vi "Convert Measurement.vi"() -> ()   [LabVIEW 2021]
uses:
  _Measurement Plugin Converter/Converter/Queue Driver/controls/Queue Operations.ctl
  _Measurement Plugin Converter/Converter/Conversion Logic/controls/Data Holder.ctl
  _Measurement Plugin Converter/Converter/Conversion Logic/controls/Input Data.ctl
  _Measurement Plugin Converter/Converter/Conversion Logic/controls/Module Data.ctl
  _Measurement Plugin Converter/Utilities/Logger Utilities/Event Logger/TypeDef/EventDataCluster.ctl
  _Measurement Plugin Converter/Utilities/Logger Utilities/Event Logger/TypeDef/EventValues.ctl
  _Measurement Plugin Converter/Converter/Converter Reusables/controls/Dictionary States.ctl
  <vilib>/Utility/cursorutil.llb/Set Cursor (Icon Pict).vi
  _Measurement Plugin Converter/Converter/Queue Driver/Queue Driver.lvlib
  _Measurement Plugin Converter/Converter/Conversion Logic/Converter.lvlib
  _Measurement Plugin Converter/Converter/Path Functions/Path Functions.lvlib
  _Measurement Plugin Converter/Converter/Converter Reusables/Converter Reusables.lvlib
  _Measurement Plugin Converter/Utilities/Logger Utilities/Event Logger/Event Logger.lvlib
  _Measurement Plugin Converter/Utilities/Sequence Creation/Create Sequence.lvlib
panel:
  out "Tab Control":enum32{"User Inputs", "Progress", "Next Steps"}(tab)
  in  "CreateSeq?":bool
  in  "Description":string caption="Measurement Plug-in Description"
  in  "Project Path":path caption="Select the Project Path"
  in  "Measurement VI":path caption="Select Measurement VI"
  in  "Plug-in Name":string caption="Measurement Plug-in Name"
  in  "Create Measurement Service":bool
  out "Warning":bool=TRUE caption="1. Measurement should be a VI\n2. Measurement plug-in name must be unique \n3. Plugin name cannot contain any of the following characters:\n         \\ / : * ? \" < > |"
  out "Progress":i8(slide) scale=0.0..100.0
  out "Status":string
  in  "Go Home":bool
  out "Launch IS":string
  out "Run Service":string
  out "Launch Type Spec":string
  out "Launch Logic":string
  out "Launch UI":string
  out "Pinmap Link":string
  out "TestStand Link":string
  out "MeasLink Link":string
  # "* Project in which the measurement plug-in will be created"
  # "Measurement Converted Successfully!"
  # "Run the Measurement:\n1. Run the measurement service. Click here to run.\n2. Launch the Template InstrumentStudio project.\n3. Add instruments and pins in PinMap.\n4. Add SoftPanel and run the measurement."
  # "Review the Measurement:\n1. Review the Measurement UI. Click here to launch.\n2. Review the Measurement Logic VI. Click here to launch.\n3. Review the Type Specialization VI. Click here to launch."
  # "Related Information:\n• InstrumentStudio Pro\n• PinMap\n• TestStand"
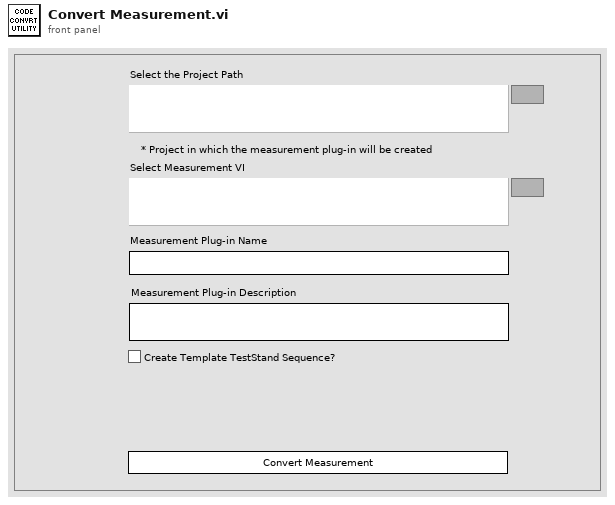
[diagram p1: front panel]
types:
  T1 = typedef "Queue Driver.lvlib/Queue Operations.ctl" = enum16{"Create Q", "Enqueue", "Enqueue N", "Dequeue", "Flush", "Release"}
  T2 = enum8{"Enabled", "Disabled", "Disabled and Grayed Out"}
  T3 = typedef "Converter.lvlib/Data Holder.ctl" = cluster{"Input Data":T4, "Module Data":T5, "TestStandAval?":bool, "EventData":T6}
  T4 = typedef "Converter.lvlib/Input Data.ctl" = cluster{"Project Path":path, "Code Module":path, "Measurement Name":string, "Description":string, "CreateSeq?":bool}
  T5 = typedef "Converter.lvlib/Module Data.ctl" = cluster{"Valid Code Path?":bool, "Valid Meas Name?":bool, "VI extension":string}
  T6 = typedef "Event Logger.lvlib/EventDataCluster.ctl" = cluster{"LoggerPath":path, "FileCount":i32, "EventValues":T7, "ExtendedFilePath":path}
  T7 = typedef "Event Logger.lvlib/EventValues.ctl" = string
  T8 = typedef "Converter Reusables.lvlib/Dictionary States.ctl" = enum16{"Set", "Get", "Delete", "Delete All"}
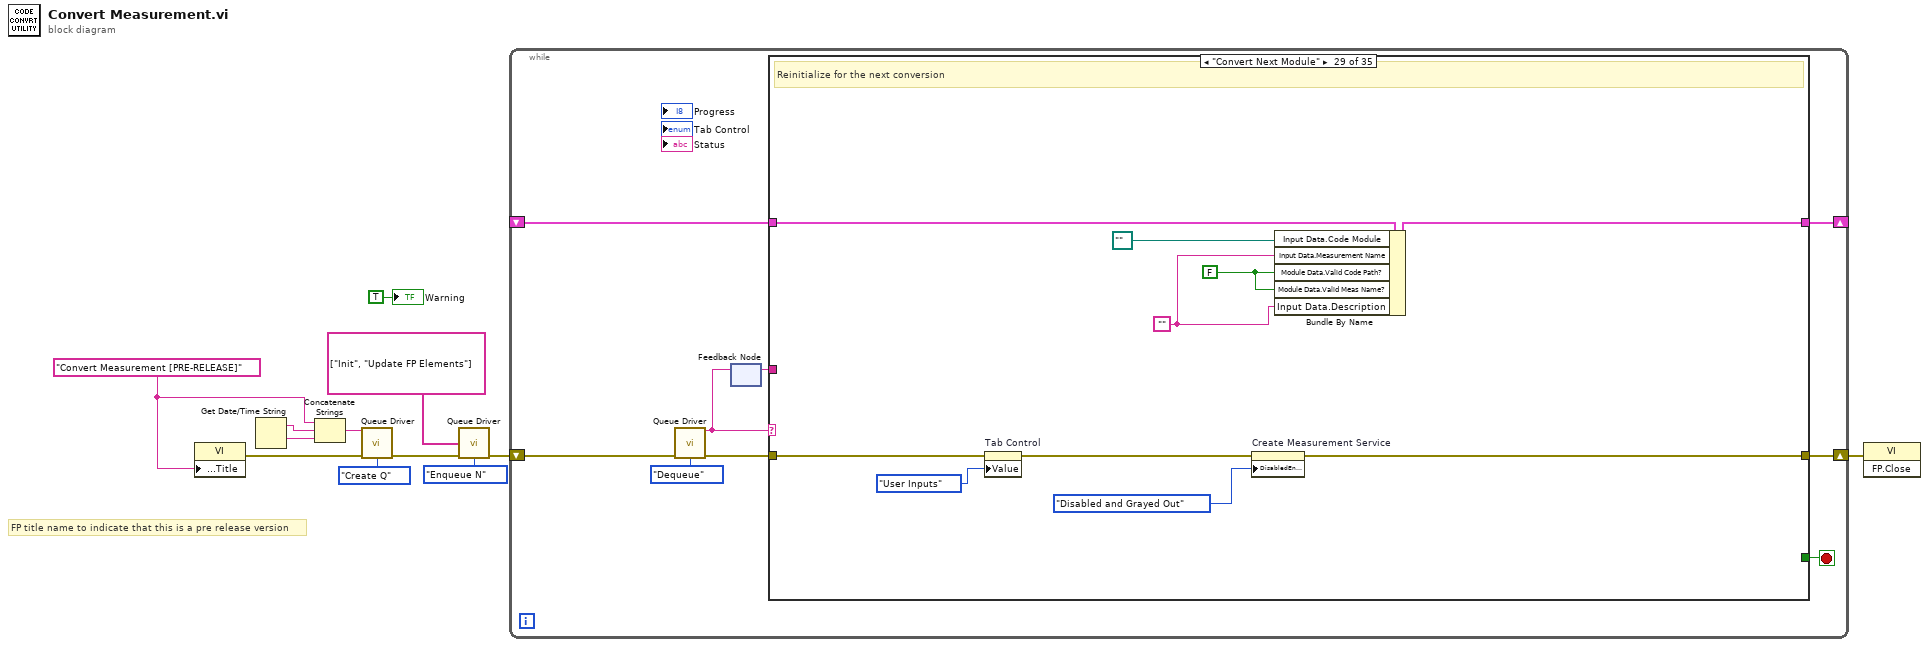
[diagram p0: block diagram]
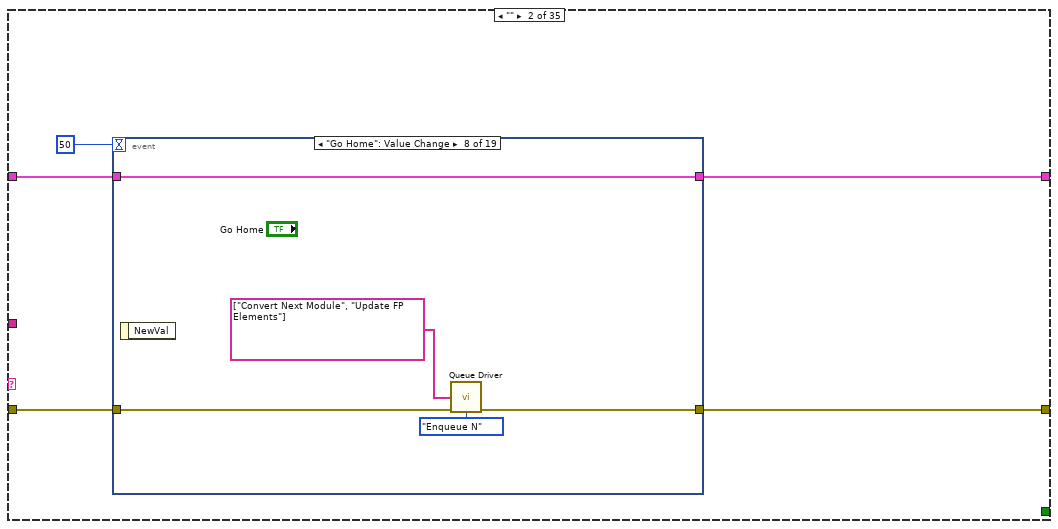
[diagram p3: hidden frame]
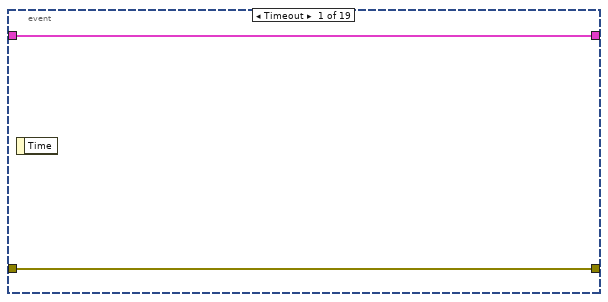
[diagram p4: hidden frame]
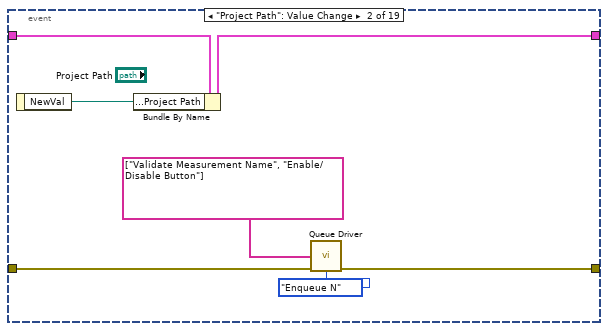
[diagram p5: hidden frame]
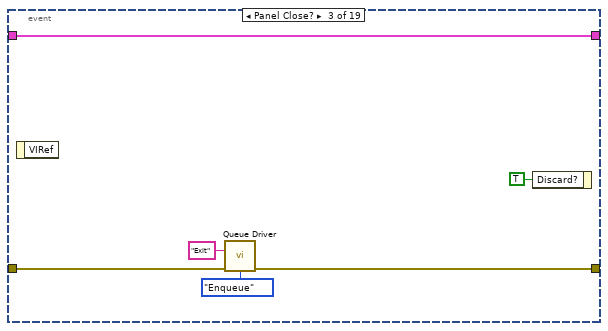
[diagram p6: hidden frame]
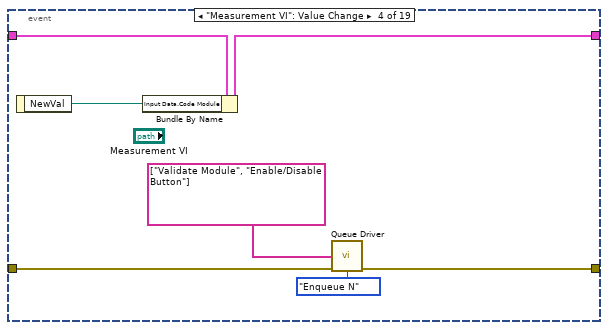
[diagram p7: hidden frame]
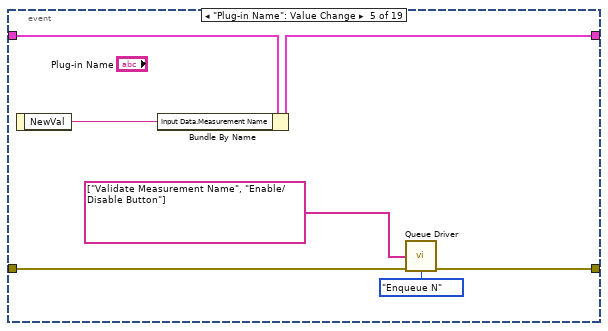
[diagram p8: hidden frame]
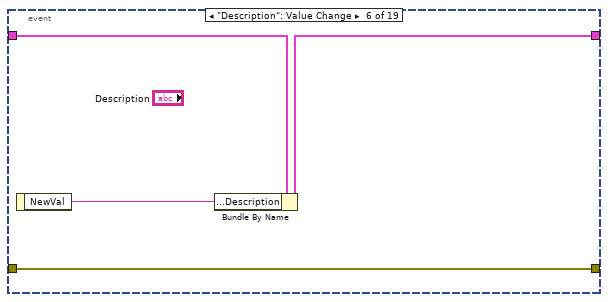
[diagram p9: hidden frame]
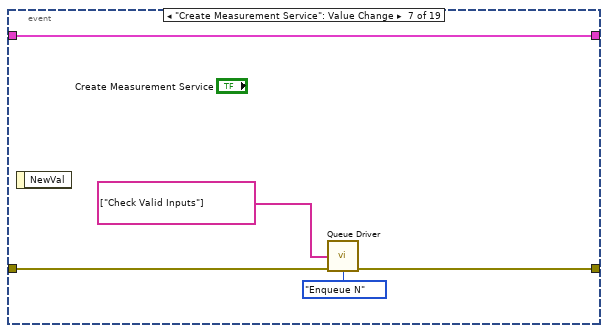
[diagram p10: hidden frame]
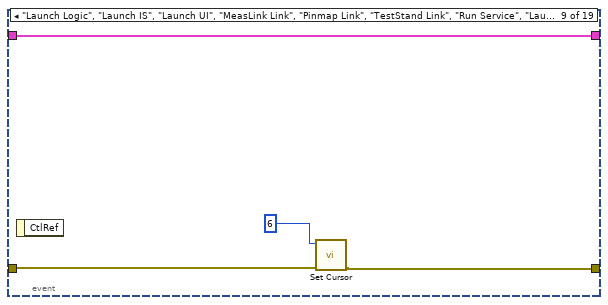
[diagram p11: hidden frame]
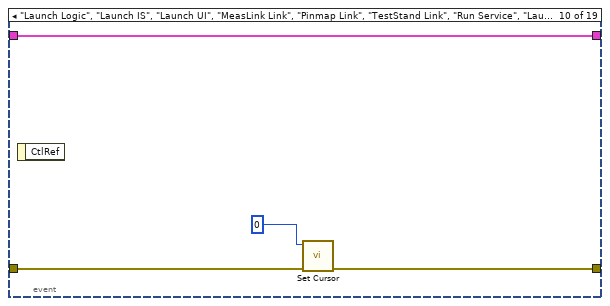
[diagram p12: hidden frame]
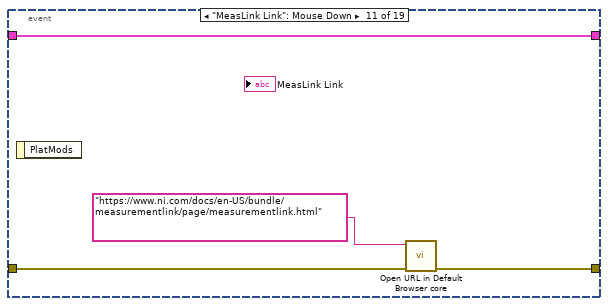
[diagram p13: hidden frame]
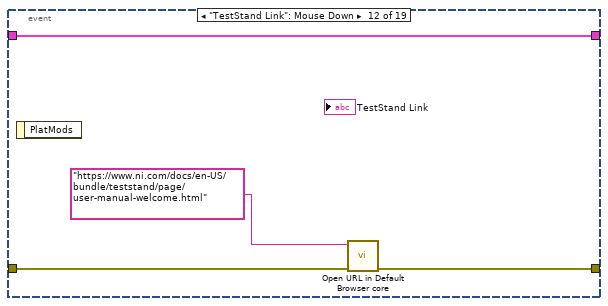
[diagram p14: hidden frame]
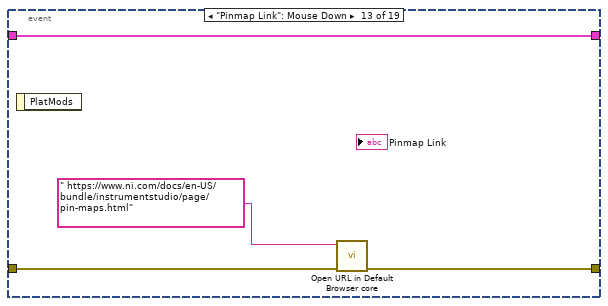
[diagram p15: hidden frame]
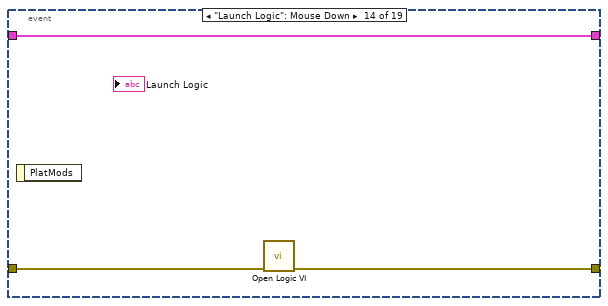
[diagram p16: hidden frame]
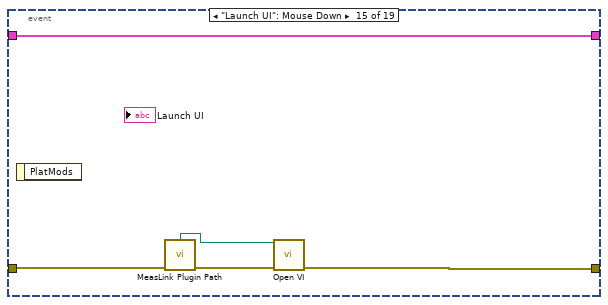
[diagram p17: hidden frame]
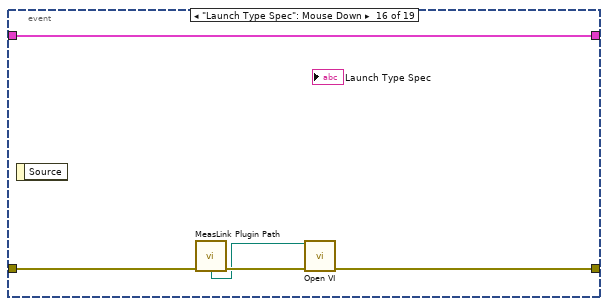
[diagram p18: hidden frame]
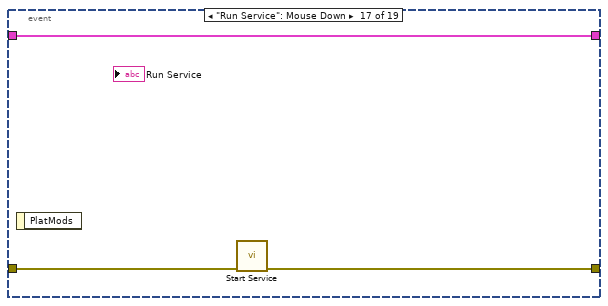
[diagram p19: hidden frame]
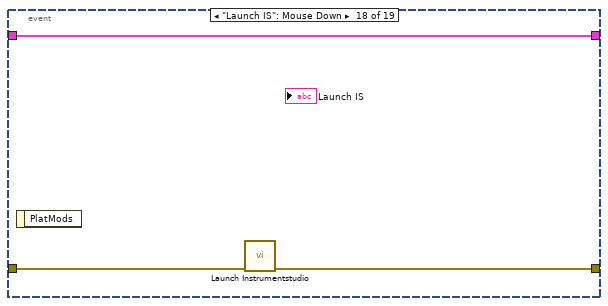
[diagram p20: hidden frame]
diagram:
  w1 = "Convert Measurement [PRE-RELEASE]" ("Front Panel Window:Title")
  # "FP title name to indicate that this is a pre release version"
  n1 = property class="VI"("Front Panel.Title"=w1) -> (error out=w2:errorcluster)  [unwired: 2 in, 1 out]
  n2 = Get Date/Time String() -> (date string=w8:string, time string=w7:string)  [unwired: 3 in]
  n3 = Concatenate Strings(w1, w8, w7) -> (w6:string)
  n4 = call "Queue Driver.vi"("Name"=w6, "error in (no error)"=w2, "Q Operations"=Queue_Operations."Create Q") -> ("error out"=w9:errorcluster)  [unwired: 11 in, 1 out]
  n5 = call "Queue Driver.vi"("States[]"=string[] ["Init", "Update FP Elements"], "error in (no error)"=w9, "Q Operations"=Queue_Operations."Enqueue N") -> ("error out"=w11:errorcluster)  [unwired: 11 in, 1 out]
  n6 = while {
    shift-right: [w18] -> w3
    shift-left: w11 -> [w20]
    shift-right: [w14] -> _
    shift-left: _ -> [w13]
    stop <- w17 stop-if-true
    n7 = call "Queue Driver.vi"("error in (no error)"=w20, "Q Operations"=Queue_Operations."Dequeue") -> ("Dequeued State"=w16:string, "error out"=w19:errorcluster)  [unwired: 12 in]
    n8 = feedback-in #1(w16) -> ()
    n9 = feedback #1() -> (w15:string)  [unwired: 1 in]
    n10 = case shown="\"Convert Next Module\"" w16 {
      tunnel: w19 -> [w23 w27 w132 w134 w146 w156 w161 w165 w188 w212 w223 w231 w245 w254 w263 w275 w285 w297 w306 w318 w329 w339 w350 w361 w373 w384 w404 w426 w437 w443 w449 w451 w459 w462 w464]
      tunnel: [w23 w26 w125 w134 w136 w151 w161 w166 w193 w211 w223 w235 w240 w253 w261 w272 w283 w294 w301 w313 w326 w337 w346 w357 w372 w383 w394 w428 w435 w443 w448 w451 w453 w462 w469] -> w18
      tunnel: [_ _ _ _ _ _ _ _ _ _ _ _ _ _ _ _ _ _ _ _ _ _ _ _ _ _ _ _ _ _ _ _ TRUE _ _] -> w17
      tunnel: w15 -> [_ _ _ _ _ _ _ _ _ _ _ _ _ _ _ _ _ _ _ _ _ _ _ _ _ _ _ _ _ _ _ _ _ _ _]
      tunnel: [w22 w25 w131 w133 w145 w159 w160 w169 w190 w216 w222 w237 w239 w252 w260 w269 w279 w290 w305 w315 w324 w335 w349 w360 w368 w380 w395 w431 w440 w442 w445 w450 w455 w461 w468] -> w14
      tunnel: w13 -> [w22 w24 _ w133 w145 w159 w160 w170 w191 w216 w222 w237 w248 w258 w267 w268 w280 w291 w311 w316 w333 w344 w355 w366 w369 w381 w403 w431 w441 w442 w447 w450 w455 w461 w468]
      frame Default {
      }
      frame "" {
        n11 = event shown="[7] \"Go Home\": Value Change" {
          selector: _ -> [_ _ _ _ _ _ _ _ _ _ _ _ _ _ _ _ _ _ _]
          dyn-events: _ -> [_ _ _ _ _ _ _ _ _ _ _ _ _ _ _ _ _ _ _]
          timeout: 50 -> [_ _ _ _ _ _ _ _ _ _ _ _ _ _ _ _ _ _ _]
          tunnel: w27 -> [w30 w32 w41 w46 w53 w61 w64 w69 w72 w76 w80 w85 w88 w92 w95 w100 w105 w108 w114]
          tunnel: [w30 w33 w40 w45 w54 w61 w65 w70 w73 w77 w81 w86 w89 w93 w96 w101 w106 w109 w114] -> w26
          tunnel: [w29 w36 w43 w49 w56 w59 w66 w71 w75 w79 w83 w87 w91 w94 w99 w104 w107 w110 w112] -> w25
          tunnel: w24 -> [w29 w37 w43 w50 w57 w60 w66 w71 w75 w79 w83 w87 w91 w94 w99 w104 w107 w110 w113]
          event Timeout {
            n12 = event-data() -> ()  [unwired: 1 in, 1 out]
          }
          event "Project Path": Value Change {
            n13 = event-data() -> ("NewVal"=w35:path)  [unwired: 1 in]
            n14 = Bundle By Name(cluster=w37, "Input Data.Project Path"=w35) -> (w36:T3)
            n15 = call "Queue Driver.vi"("States[]"=string[] ["Validate Measurement Name", "Enable/Disable Button"], "error in (no error)"=w32, "Q Operations"=Queue_Operations."Enqueue N") -> ("error out"=w33:errorcluster)  [unwired: 11 in, 1 out]
          }
          event Panel Close? {
            n16 = event-data() -> ()  [unwired: 1 in, 1 out]
            n17 = call "Queue Driver.vi"("State"="Exit", "error in (no error)"=w41, "Q Operations"=Queue_Operations."Enqueue") -> ("error out"=w40:errorcluster)  [unwired: 11 in, 1 out]
            n18 = event-data("Discard?"=TRUE) -> ()  [unwired: 1 in, 1 out]
          }
          event "Measurement VI": Value Change {
            n19 = event-data() -> ("NewVal"=w48:path)  [unwired: 1 in]
            n20 = Bundle By Name(cluster=w50, "Input Data.Code Module"=w48) -> (w49:T3)
            n21 = call "Queue Driver.vi"("States[]"=string[] ["Validate Module", "Enable/Disable Button"], "error in (no error)"=w46, "Q Operations"=Queue_Operations."Enqueue N") -> ("error out"=w45:errorcluster)  [unwired: 11 in, 1 out]
          }
          event "Plug-in Name": Value Change {
            n22 = event-data() -> ("NewVal"=w55:string)  [unwired: 1 in]
            n23 = Bundle By Name(cluster=w57, "Input Data.Measurement Name"=w55) -> (w56:T3)
            n24 = call "Queue Driver.vi"("States[]"=string[] ["Validate Measurement Name", "Enable/Disable Button"], "error in (no error)"=w53, "Q Operations"=Queue_Operations."Enqueue N") -> ("error out"=w54:errorcluster)  [unwired: 11 in, 1 out]
          }
          event "Description": Value Change {
            n25 = event-data() -> ("NewVal"=w58:string)  [unwired: 1 in]
            n26 = Bundle By Name(cluster=w60, "Input Data.Description"=w58) -> (w59:T3)
          }
          event "Create Measurement Service": Value Change {
            n27 = event-data() -> ()  [unwired: 1 in, 1 out]
            n28 = call "Queue Driver.vi"("States[]"=string[] ["Check Valid Inputs"], "error in (no error)"=w64, "Q Operations"=Queue_Operations."Enqueue N") -> ("error out"=w65:errorcluster)  [unwired: 11 in, 1 out]
          }
          event "Go Home": Value Change {
            n29 = event-data() -> ()  [unwired: 1 in, 1 out]
            n30 = call "Queue Driver.vi"("States[]"=string[] ["Convert Next Module", "Update FP Elements"], "error in (no error)"=w69, "Q Operations"=Queue_Operations."Enqueue N") -> ("error out"=w70:errorcluster)  [unwired: 11 in, 1 out]
          }
          event "Launch Logic", "Launch IS", "Launch UI", "MeasLink Link", "Pinmap Link", "TestStand Link", "Run Service", "Launch Type Spec": Mouse Enter {
            n31 = event-data() -> ()  [unwired: 1 in, 1 out]
            n32 = call-poly <vilib>:"Set Cursor.vi"("error in (no error)"=w72, "icon"=u16 6) -> ("error out"=w73:errorcluster)  [unwired: 8 in, 1 out]
          }
          event "Launch Logic", "Launch IS", "Launch UI", "MeasLink Link", "Pinmap Link", "TestStand Link", "Run Service", "Launch Type Spec": Mouse Leave {
            n33 = event-data() -> ()  [unwired: 1 in, 1 out]
            n34 = call-poly <vilib>:"Set Cursor.vi"("error in (no error)"=w76, "icon"=u16 0) -> ("error out"=w77:errorcluster)  [unwired: 8 in, 1 out]
          }
          event "MeasLink Link": Mouse Down {
            n35 = event-data() -> ()  [unwired: 1 in, 1 out]
            n36 = call <vilib>:"Open URL in Default Browser core.vi"("error in (no error)"=w80, "url"="https://www.ni.com/docs/en-US/bundle/measurementlink/page/measurementlink.html" ("URL")) -> ("error out"=w81:errorcluster)  [unwired: 4 in, 1 out]
          }
          event "TestStand Link": Mouse Down {
            n37 = event-data() -> ()  [unwired: 1 in, 1 out]
            n38 = call <vilib>:"Open URL in Default Browser core.vi"("error in (no error)"=w85, "url"="https://www.ni.com/docs/en-US/bundle/teststand/page/user-manual-welcome.html" ("URL")) -> ("error out"=w86:errorcluster)  [unwired: 4 in, 1 out]
          }
          event "Pinmap Link": Mouse Down {
            n39 = event-data() -> ()  [unwired: 1 in, 1 out]
            n40 = call <vilib>:"Open URL in Default Browser core.vi"("error in (no error)"=w88, "url"=" https://www.ni.com/docs/en-US/bundle/instrumentstudio/page/pin-maps.html" ("URL")) -> ("error out"=w89:errorcluster)  [unwired: 4 in, 1 out]
          }
          event "Launch Logic": Mouse Down {
            n41 = event-data() -> ()  [unwired: 1 in, 1 out]
            n42 = call "Open Logic VI.vi"("error in (no error)"=w92) -> ("error out"=w93:errorcluster)  [unwired: 14 in]
          }
          event "Launch UI": Mouse Down {
            n43 = event-data() -> ()  [unwired: 1 in, 1 out]
            n44 = call "MeasLink Plugin Path.vi"("error in (no error)"=w95) -> ("Measurement UI"=w97:path, "error out"=w98:errorcluster)  [unwired: 2 in, 11 out]
            n45 = call "Open VI.vi"("Logic VI Path"=w97, "error in (no error)"=w98) -> ("error out"=w96:errorcluster)  [unwired: 13 in]
          }
          event "Launch Type Spec": Mouse Down {
            n46 = event-data() -> ()  [unwired: 1 in, 1 out]
            n47 = call "MeasLink Plugin Path.vi"("error in (no error)"=w100) -> ("Type Specialization"=w102:path, "error out"=w103:errorcluster)  [unwired: 2 in, 11 out]
            n48 = call "Open VI.vi"("Logic VI Path"=w102, "error in (no error)"=w103) -> ("error out"=w101:errorcluster)  [unwired: 13 in]
          }
          event "Run Service": Mouse Down {
            n49 = event-data() -> ()  [unwired: 1 in, 1 out]
            n50 = call "Start Service.vi"("error in (no error)"=w105) -> ("error out"=w106:errorcluster)  [unwired: 14 in]
          }
          event "Launch IS": Mouse Down {
            n51 = event-data() -> ()  [unwired: 1 in, 1 out]
            n52 = call "Launch Instrumentstudio.vi"("error in (no error)"=w108) -> ("error out"=w109:errorcluster)  [unwired: 14 in]
          }
          event "CreateSeq?": Value Change {
            n53 = event-data() -> ("NewVal"=w111:bool)  [unwired: 1 in]
            n54 = Bundle By Name(cluster=w113, "Input Data.CreateSeq?"=w111) -> (w112:T3)
          }
        }
      }
      frame "Init" {
        # "Initilialize the Data and the UI Data"
        n55 = call "Get Default Project Path.vi"("error in"=w132) -> ("Project Path"=w130:path, "error out"=w128:errorcluster)  [unwired: 13 in]
        n56 = property on="Warning" class="Bool"(error in=w128, "Visible"=FALSE) -> (error out=w126:errorcluster)  [unwired: 1 in, 1 out]
        n57 = property on="Create Measurement Service" class="Bool"(error in=w126, "DisabledEnum"=T2."Disabled and Grayed Out" ("Disabled")) -> (error out=w123:errorcluster)  [unwired: 1 in, 1 out]
        n58 = call "VerifyTestStandAvailability.vi"("Error In"=w123) -> ("TestStandInstalled?"=w116:bool, "Error Out"=w122:errorcluster)  [unwired: 13 in]
        n59 = call "CreateLogFile.vi"("Error In"=w122) -> ("EventDataOut"=w117:T6, "Error Out"=w124:errorcluster)  [unwired: 13 in]
        n60 = property on="CreateSeq?" class="Bool (strict)"(error in=w124, "Value"=w116) -> (error out=w125:errorcluster)  [unwired: 1 in, 1 out]
        n61 = Bundle By Name(cluster=T3 {"Input Data"={"Project Path"=path "", "Code Module"=path "", "Measurement Name"="", "Description"="", "CreateSeq?"=FALSE}, "Module Data"={"Valid Code Path?"=FALSE, "Valid Meas Name?"=FALSE, "VI extension"=""}, "TestStandAval?"=FALSE, "EventData"={"LoggerPath"=path "", "FileCount"=0, "EventValues"="", "ExtendedFilePath"=path ""}} ("Data Holder"), "Input Data.Project Path"=w130, "Input Data.Code Module"=path "", "Input Data.Measurement Name"="", "Module Data.VI extension"="vi" ("Input Data.Measurement Name"), "TestStandAval?"=w116, "Input Data.CreateSeq?"=w116, "EventData"=w117, "Input Data.Description"="") -> (w131:T3)
      }
      frame "*********************FRONT PANEL RELATED****************" {
      }
      frame "Update FP Elements" {
        # "Update the Front Panel Elements"
        n62 = Unbundle By Name(w145) -> ("Input Data.Description"=w137:string, "TestStandAval?"=w139:bool, "Input Data.Measurement Name"=w142:string, "Input Data.Code Module"=w143:path, "Input Data.Project Path"=w144:path)
        n63 = property on="Project Path" class="Path"(error in=w146, "Value"=w144) -> (error out=w148:errorcluster)  [unwired: 1 in, 1 out]
        n64 = property on="Measurement VI" class="Path"(error in=w148, "Value"=w143) -> (error out=w147:errorcluster)  [unwired: 1 in, 1 out]
        n65 = property on="Plug-in Name" class="Str"(error in=w147, "Value"=w142) -> (error out=w140:errorcluster)  [unwired: 1 in, 1 out]
        n66 = property on="Tab Control" class="TabCtl (strict)"(error in=w140, "Value"=enum32{"User Inputs", "Progress", "Next Steps"}."User Inputs" ("Tab Control")) -> (error out=w138:errorcluster)  [unwired: 1 in, 1 out]
        n67 = property on="CreateSeq?" class="Bool (strict)"(error in=w138, "Visible"=w139) -> (error out=w135:errorcluster)  [unwired: 1 in, 1 out]
        n68 = property on="Description" class="Str"(error in=w135, "Value"=w137) -> (error out=w136:errorcluster)  [unwired: 1 in, 1 out]
      }
      frame "Enable/Disable Button" {
        n69 = Unbundle By Name(w159) -> ("Module Data.Valid Code Path?"=w158:bool, "Module Data.Valid Meas Name?"=w157:bool)
        n70 = And(x=w158, y=w157) -> (x .and. y?=w152:bool)
        n71 = Select(t=T2."Enabled" ("Disabled"), s=w152, f=T2."Disabled and Grayed Out" ("Disabled")) -> (s? t:f=w153:T2)
        n72 = property on="Create Measurement Service" class="Bool"(error in=w156, "DisabledEnum"=w153) -> (error out=w150:errorcluster)  [unwired: 1 in, 1 out]
        n73 = Not(x=w152) -> (.not. x?=w149:bool)
        n74 = property on="Warning" class="Bool"(error in=w150, "Visible"=w149) -> (error out=w151:errorcluster)  [unwired: 1 in, 1 out]
      }
      frame "**********************INPUT VALIDATION******************" {
      }
      frame "Validate Measurement Name" {
        n75 = Unbundle By Name(w170) -> ("Input Data.Project Path"=w172:path, "Input Data.Measurement Name"=w171:string)
        n76 = call "Set Cursor Icon.vi"("Cursor Icon"=u16 2, "error in (no error)"=w165) -> ("error out"=w164:errorcluster)  [unwired: 13 in]
        n77 = Empty String/Path?(string/path=w172) -> (empty?=w162:bool)
        n78 = case "Valid Path and Name ?" shown="False" w162 {
          tunnel: w164 -> [w181 w183]
          tunnel: w172 -> [w180 _]
          tunnel: w171 -> [w179 _]
          tunnel: [w176 w183] -> w167
          tunnel: w170 -> [w175 w182]
          tunnel: [w174 w182] -> w169
          frame False {
            # "Validate the Path and Measurement Name"
            n79 = call "Valiadate Plugin Name.vi"("Path"=w180, "library name"=w179, "error in (no error)"=w181) -> ("Valid Name?"=w173:bool, "error out"=w177:errorcluster)  [unwired: 11 in]
            n80 = Not(x=w173) -> (.not. x?=w178:bool)
            n81 = Bundle By Name(cluster=w175, "Module Data.Valid Meas Name?"=w173) -> (w174:T3)
            n82 = property on="Warning" class="Bool"(error in=w177, "Visible"=w178) -> (error out=w176:errorcluster)  [unwired: 1 in, 1 out]
          }
          frame True {
          }
        }
        n83 = call "Set Cursor Icon.vi"("Cursor Icon"=u16 0 ("icon"), "error in (no error)"=w167) -> ("error out"=w166:errorcluster)  [unwired: 13 in]
      }
      frame "Validate Module" {
        # "Validate the Module Extension"
        n84 = Unbundle By Name(w191) -> ("Module Data.VI extension"=w195:string, "Input Data.Code Module"=w184:path)
        n85 = call <vilib>:"Check if File or Folder Exists.vi"("error in (no error)"=w188, "path"=w184) -> ("error out"=w189:errorcluster, "file or folder exists?"=w186:bool)  [unwired: 7 in, 1 out]
        n86 = call <vilib>:"Get File Extension.vi"("error in (no error)"=w189, "file"=w184) -> ("error out"=w194:errorcluster, "filename without extension"=w192:string, "lowercase file extension"=w196:string)  [unwired: 5 in, 2 out]
        n87 = Equal?(x=w195, y=w196) -> (x = y?=w187:bool)
        n88 = And(x=w186, y=w187) -> (x .and. y?=w185:bool)
        n89 = case shown="True" w185 {
          selector: w185 -> [w200 w203]
          tunnel: w194 -> [w199 w210]
          tunnel: [w198 w207] -> w193
          tunnel: w192 -> [_ w204]
          tunnel: w191 -> [w202 w206]
          tunnel: [w201 w205] -> w190
          frame False {
            n90 = property on="Warning" class="Bool"(error in=w199, "Visible"=TRUE) -> (error out=w198:errorcluster)  [unwired: 1 in, 1 out]
            n91 = Bundle By Name(cluster=w202, "Module Data.Valid Code Path?"=w200) -> (w201:T3)
          }
          frame True {
            n92 = Not(x=w203) -> (.not. x?=w209:bool)
            n93 = property on="Warning" class="Bool"(error in=w210, "Visible"=w209) -> (error out=w208:errorcluster)  [unwired: 1 in, 1 out]
            n94 = Bundle By Name(cluster=w206, "Module Data.Valid Code Path?"=w203, "Input Data.Measurement Name"=w204) -> (w205:T3)
            n95 = property on="Plug-in Name" class="Str"(error in=w208, "Val(Sgnl)"=w204) -> (error out=w207:errorcluster)  [unwired: 1 in, 1 out]
          }
        }
      }
      frame "Check Valid Inputs" {
        # "Check if all the inputs are valid and start conversion"
        n96 = Unbundle By Name(w216) -> ("Module Data.Valid Code Path?"=w215:bool, "Module Data.Valid Meas Name?"=w214:bool)
        n97 = And(x=w215, y=w214) -> (x .and. y?=w213:bool)
        n98 = case "Valid Inputs?" shown="True" w213 {
          tunnel: w212 -> [w217 w220]
          tunnel: [w217 w219] -> w211
          frame False {
          }
          frame True {
            n99 = call "Queue Driver.vi"("States[]"=string[] ["Init Conversion", "Check if Project exists", "Event Logger", "Add VI to library", "Event Logger", "Get Driver List", "Event Logger", "Edit Input Controls", "Edit Result Controls", "Edit Module Connector Pane", "Event Logger", "Create Wrapper", "Deserialize Cluster Data", "Add MeasLink APIs", "Event Logger", "Disable Initialize APIs", "Event Logger", "Edit Type Specialization", "Event Logger", "Add UI Elements", "Event Logger", "Flatten the Clusters", "Event Logger", "Handling Default Value", "Event Logger", "Create Sequence", "Event Logger", "Show Next Steps"], "error in (no error)"=w220, "Q Operations"=Queue_Operations."Enqueue N") -> ("error out"=w219:errorcluster)  [unwired: 11 in, 1 out]
          }
        }
      }
      frame "**********************CODE CONVERSION**********************" {
      }
      frame "Init Conversion" {
        # "Init Code Conversion by setting the value in Dictionaries"
        n100 = property on="Status" class="Str"(error in=w231, "Value"="Initializing Conversion..." ("Status")) -> (error out=w233:errorcluster)  [unwired: 1 in, 1 out]
        n101 = Unbundle By Name(w237) -> ("Input Data.Code Module"=w226:path, "Input Data.Project Path"=w228:path, "Input Data.Measurement Name"=w230:string)
        n102 = property on="Progress" class="Slide (strict)"(error in=w233, "Value"=i8 2 ("Progress")) -> (error out=w229:errorcluster)  [unwired: 1 in, 1 out]
        n103 = call "Set Measurement Name.vi"("Name"=w230, "error in (no error)"=w229) -> ("error out"=w227:errorcluster)  [unwired: 13 in]
        n104 = call "Set Project Path.vi"("Project Path"=w228, "error in (no error)"=w227) -> ("error out"=w225:errorcluster)  [unwired: 13 in]
        n105 = call "Set Code Module Path.vi"("CodeModule Path"=w226, "error in (no error)"=w225) -> ("error out"=w234:errorcluster)  [unwired: 13 in]
        n106 = property on="Tab Control" class="TabCtl (strict)"(error in=w234, "Value"=enum32{"User Inputs", "Progress", "Next Steps"}."Progress" ("Tab Control")) -> (error out=w235:errorcluster)  [unwired: 1 in, 1 out]
      }
      frame "Check if Project exists" {
        # "Check if project exists and create a new one"
        n107 = property on="Status" class="Str"(error in=w245, "Value"="Creating Measurement Plugin..." ("Status")) -> (error out=w242:errorcluster)  [unwired: 1 in, 1 out]
        n108 = property on="Progress" class="Slide (strict)"(error in=w242, "Value"=i8 6 ("Progress")) -> (error out=w243:errorcluster)  [unwired: 1 in, 1 out]
        n109 = Unbundle By Name(w248) -> ("Input Data.Project Path"=w247:path, "Input Data.Description"=w241:string)
        n110 = call "Project_and_Mlink Template Creation.vi"("Project Path"=w247, "Description"=w241, "error in (no error)"=w243) -> ("error out"=w240:errorcluster)  [unwired: 12 in]
        n111 = Bundle By Name(cluster=w248, "EventData.EventValues"=T7 "Create Measurement Plugin Template" ("EventValues")) -> (w239:T3)
      }
      frame "Add VI to library" {
        # "Add the code module to MeasLink Library"
        n112 = property on="Status" class="Str"(error in=w254, "Value"="Copying Measurement VI along with dependecies and adding in the project..." ("Status")) -> (error out=w257:errorcluster)  [unwired: 1 in, 1 out]
        n113 = Bundle By Name(cluster=w258, "EventData.EventValues"=T7 "Convert the MeasurementVI along with dependencies" ("EventValues")) -> (w252:T3)
        n114 = property on="Progress" class="Slide (strict)"(error in=w257, "Value"=i8 16 ("Progress")) -> (error out=w250:errorcluster)  [unwired: 1 in, 1 out]
        n115 = call "Copy Set Default Value VI.vi"("error in (no error)"=w250) -> ("error out"=w249:errorcluster)  [unwired: 14 in]
        n116 = call "Add VI to lib.vi"("error in"=w249) -> ("error out"=w253:errorcluster)  [unwired: 14 in]
      }
      frame "Get Driver List" {
        # "Get the list of drivers used in the Measurement VI"
        n117 = property on="Status" class="Str"(error in=w263, "Value"="Fetching the list of instrument drivers used..." ("Status")) -> (error out=w266:errorcluster)  [unwired: 1 in, 1 out]
        n118 = property on="Progress" class="Slide (strict)"(error in=w266, "Value"=i8 20 ("Progress")) -> (error out=w262:errorcluster)  [unwired: 1 in, 1 out]
        n119 = Bundle By Name(cluster=w267, "EventData.EventValues"=T7 "Get the list of drivers used in the Measurement VI" ("EventValues")) -> (w260:T3)
        n120 = call "Driver Lists.vi"("error in (no error)"=w262) -> ("error out"=w261:errorcluster)  [unwired: 14 in]
      }
      frame "Edit Input Controls" {
        # "Add elements in the Measurement Configuration.ctl"
        n121 = property on="Status" class="Str"(error in=w275, "Value"="Editing Measurement Configuration..." ("Status")) -> (error out=w278:errorcluster)  [unwired: 1 in, 1 out]
        n122 = property on="Progress" class="Slide (strict)"(error in=w278, "Value"=i8 24 ("Progress")) -> (error out=w274:errorcluster)  [unwired: 1 in, 1 out]
        n123 = call "Add MeasLink Controls.vi"("error in (no error)"=w274) -> ("error out"=w273:errorcluster)  [unwired: 14 in]
        n124 = Bundle By Name(cluster=w268, "EventData.EventValues"=T7 "Edit the input output configuration of copied Measurement VI" ("EventValues")) -> (w269:T3)
        n125 = call "Set SubroutineInfo.vi"("Subroutine In"="Add controls from Measurement VI to Measurement Configuration.ctl", "error in (no error)"=w273) -> ("error out"=w272:errorcluster)  [unwired: 13 in]
      }
      frame "Edit Result Controls" {
        # "Add elements in the Measurement Results.ctl"
        n126 = property on="Status" class="Str"(error in=w285, "Value"="Editing Measurement Results..." ("Status")) -> (error out=w288:errorcluster)  [unwired: 1 in, 1 out]
        n127 = property on="Progress" class="Slide (strict)"(error in=w288, "Value"=i8 28 ("Progress")) -> (error out=w284:errorcluster)  [unwired: 1 in, 1 out]
        n128 = call "Add MeasLink Indicators.vi"("error in (no error)"=w284) -> ("error out"=w289:errorcluster)  [unwired: 14 in]
        n129 = Bundle By Name(cluster=w280, "EventData.EventValues"=T7 "Editing the results control" ("EventValues")) -> (w279:T3)
        n130 = call "Set SubroutineInfo.vi"("Subroutine In"="Add indicators from Measurement VI to Measurement Results.ctl", "error in (no error)"=w289) -> ("error out"=w283:errorcluster)  [unwired: 13 in]
      }
      frame "Edit Module Connector Pane" {
        # "Edit the connector pane of the duplicate code module"
        n131 = property on="Status" class="Str"(error in=w297, "Value"="Editing the Connector Pane of the Measurement.." ("Status")) -> (error out=w300:errorcluster)  [unwired: 1 in, 1 out]
        n132 = property on="Progress" class="Slide (strict)"(error in=w300, "Value"=i8 34 ("Progress")) -> (error out=w295:errorcluster)  [unwired: 1 in, 1 out]
        n133 = Bundle By Name(cluster=w291, "EventData.EventValues"=T7 "Editing the connector pane of the measurement" ("EventValues")) -> (w290:T3)
        n134 = call "Edit Connector Pane.vi"("error in (no error)"=w295) -> ("error out"=w296:errorcluster)  [unwired: 14 in]
        n135 = call "Set SubroutineInfo.vi"("Subroutine In"="Editing connector pane configuration of copied measurement VI", "error in (no error)"=w296) -> ("error out"=w294:errorcluster)  [unwired: 13 in]
      }
      frame "Create Wrapper" {
        # "Create a wrapper for the code module which will be placed in the Core Logic.vi"
        n136 = property on="Status" class="Str"(error in=w306, "Value"="Creating Wrapper for the Measurement..." ("Status")) -> (error out=w310:errorcluster)  [unwired: 1 in, 1 out]
        n137 = property on="Progress" class="Slide (strict)"(error in=w310, "Value"=i8 40 ("Progress")) -> (error out=w307:errorcluster)  [unwired: 1 in, 1 out]
        n138 = Bundle By Name(cluster=w311, "EventData.EventValues"=T7 "Creating wrapper for the measurement" ("EventValues")) -> (w305:T3)
        n139 = call "Create Wrapper for Code Module.vi"("error in (no error)"=w307) -> ("error out"=w302:errorcluster)  [unwired: 14 in]
        n140 = call "Set SubroutineInfo.vi"("Subroutine In"="Creating wrapper for the measurement", "error in (no error)"=w302) -> ("error out"=w301:errorcluster)  [unwired: 13 in]
      }
      frame "Deserialize Cluster Data" {
        # "Create a wrapper for the code module which will be placed in the Core Logic.vi"
        n141 = property on="Status" class="Str"(error in=w318, "Value"="Flattening and Unflattening the cluster data in Wrapper..." ("Status")) -> (error out=w322:errorcluster)  [unwired: 1 in, 1 out]
        n142 = property on="Progress" class="Slide (strict)"(error in=w322, "Value"=i8 46 ("Progress")) -> (error out=w319:errorcluster)  [unwired: 1 in, 1 out]
        n143 = call "Deserialize Connections in Wrapper.vi"("error in (no error)"=w319) -> ("error out"=w312:errorcluster)  [unwired: 14 in]
        n144 = Bundle By Name(cluster=w316, "EventData.EventValues"=T7 "Deserialize cluster elements in Logic" ("EventValues")) -> (w315:T3)
        n145 = call "Set SubroutineInfo.vi"("Subroutine In"="Deserialize the cluster data in the logic", "error in (no error)"=w312) -> ("error out"=w313:errorcluster)  [unwired: 13 in]
      }
      frame "Add MeasLink APIs" {
        # "Add all the rquired MeasLink APIs in Core Logic.vi and wire them appropriately"
        n146 = property on="Status" class="Str"(error in=w329, "Value"="Editing Measurement Logic VI..." ("Status")) -> (error out=w332:errorcluster)  [unwired: 1 in, 1 out]
        n147 = property on="Progress" class="Slide (strict)"(error in=w332, "Value"=i8 56 ("Progress")) -> (error out=w328:errorcluster)  [unwired: 1 in, 1 out]
        n148 = call "Create ML subVIs.vi"("error in (no error)"=w328) -> ("error out"=w327:errorcluster)  [unwired: 14 in]
        n149 = Bundle By Name(cluster=w333, "EventData.EventValues"=T7 "Add Session Manager APIs to the Measurement Logic" ("EventValues")) -> (w324:T3)
        n150 = call "Set SubroutineInfo.vi"("Subroutine In"="Add Session Manager APIs to the Measurement Logic", "error in (no error)"=w327) -> ("error out"=w326:errorcluster)  [unwired: 13 in]
      }
      frame "Disable Initialize APIs" {
        # "Disable the initialize and close in the code module"
        n151 = property on="Status" class="Str"(error in=w339, "Value"="Disabling and removing the Initalize and Close APIs.." ("Status")) -> (error out=w343:errorcluster)  [unwired: 1 in, 1 out]
        n152 = property on="Progress" class="Slide (strict)"(error in=w343, "Value"=i8 66 ("Progress")) -> (error out=w340:errorcluster)  [unwired: 1 in, 1 out]
        n153 = call "Add Diagram disable structure.vi"("error in (no error)"=w340) -> ("error out"=w338:errorcluster)  [unwired: 14 in]
        n154 = Bundle By Name(cluster=w344, "EventData.EventValues"=T7 "Disable Initialize and Close driver APIs") -> (w335:T3)
        n155 = call "Set SubroutineInfo.vi"("Subroutine In"="Disable the Initilalize and Close API present in the code module", "error in (no error)"=w338) -> ("error out"=w337:errorcluster)  [unwired: 13 in]
      }
      frame "Edit Type Specialization" {
        # "Edit the Type Specializations.vi"
        n156 = property on="Status" class="Str"(error in=w350, "Value"="Editing the Type Specialization VI..." ("Status")) -> (error out=w354:errorcluster)  [unwired: 1 in, 1 out]
        n157 = property on="Progress" class="Slide (strict)"(error in=w354, "Value"=i8 70 ("Progress")) -> (error out=w351:errorcluster)  [unwired: 1 in, 1 out]
        n158 = call "Edit Type Specialization.vi"("error in (no error)"=w351) -> ("error out"=w347:errorcluster)  [unwired: 14 in]
        n159 = Bundle By Name(cluster=w355, "EventData.EventValues"=T7 "Edit the Type Specialization VI") -> (w349:T3)
        n160 = call "Set SubroutineInfo.vi"("Subroutine In"="Map the Pin names in the type specialization", "error in (no error)"=w347) -> ("error out"=w346:errorcluster)  [unwired: 13 in]
      }
      frame "Add UI Elements" {
        # "Edit the Measurement UI.vi"
        n161 = property on="Status" class="Str"(error in=w361, "Value"="Editing Measurement UI..." ("Status")) -> (error out=w365:errorcluster)  [unwired: 1 in, 1 out]
        n162 = property on="Progress" class="Slide (strict)"(error in=w365, "Value"=i8 74 ("Progress")) -> (error out=w362:errorcluster)  [unwired: 1 in, 1 out]
        n163 = call "Add Elements to MeasLink UI.vi"("error in (no error)"=w362) -> ("error out"=w358:errorcluster)  [unwired: 14 in]
        n164 = Bundle By Name(cluster=w366, "EventData.EventValues"=T7 "Update Measurement UI with code module's UI") -> (w360:T3)
        n165 = call "Set SubroutineInfo.vi"("Subroutine In"="Update measurement UI ", "error in (no error)"=w358) -> ("error out"=w357:errorcluster)  [unwired: 13 in]
      }
      frame "Flatten the Clusters" {
        n166 = property on="Status" class="Str"(error in=w373, "Value"="Creating events and flatten the data..." ("Status")) -> (error out=w377:errorcluster)  [unwired: 1 in, 1 out]
        n167 = property on="Progress" class="Slide (strict)"(error in=w377, "Value"=i8 78 ("Progress")) -> (error out=w371:errorcluster)  [unwired: 1 in, 1 out]
        n168 = call "Create String and Serialize Cluster Data.vi"("error in (no error)"=w371) -> ("error out"=w370:errorcluster)  [unwired: 14 in]
        n169 = Bundle By Name(cluster=w369, "EventData.EventValues"=T7 "Flattening the cluster data to string") -> (w368:T3)
        n170 = call "Set SubroutineInfo.vi"("Subroutine In"="Cluster flattening and unflattening in Measurement UI", "error in (no error)"=w370) -> ("error out"=w372:errorcluster)  [unwired: 13 in]
      }
      frame "Handling Default Value" {
        n171 = property on="Status" class="Str"(error in=w384, "Value"="Loading values for string controls in UI..." ("Status")) -> (error out=w388:errorcluster)  [unwired: 1 in, 1 out]
        n172 = property on="Progress" class="Slide (strict)"(error in=w388, "Value"=i8 82 ("Progress")) -> (error out=w382:errorcluster)  [unwired: 1 in, 1 out]
        n173 = call "Logic for Default Case.vi"("error in (no error)"=w382) -> ("error out"=w379:errorcluster)  [unwired: 14 in]
        n174 = Bundle By Name(cluster=w381, "EventData.EventValues"=T7 "Setting default values for cluster string") -> (w380:T3)
        n175 = call "Set SubroutineInfo.vi"("Subroutine In"="Setting default value for cluster based string controls", "error in (no error)"=w379) -> ("error out"=w383:errorcluster)  [unwired: 13 in]
      }
      frame "Create Sequence" {
        # "Create sample teststand sequence"
        n176 = Unbundle By Name(w403) -> ("Input Data.Project Path"=w402:path, "Input Data.Measurement Name"=w401:string, "Input Data.CreateSeq?"=w398:bool)
        n177 = Select(t="Creating Template TestStand Measurement Sequence..." ("Status"), s=w398, f="Skipping Template Measurement Sequence Creation...") -> (s? t:f=w397:string)
        n178 = Current VI's Path() -> (path=w392:path)
        n179 = property on="Status" class="Str"(error in=w404, "Value"=w397) -> (error out=w406:errorcluster)  [unwired: 1 in, 1 out]
        n180 = Strip Path(path=w392) -> (stripped path=w391:path)  [unwired: 1 out]
        n181 = property on="Progress" class="Slide (strict)"(error in=w406, "Value"=i8 90 ("Progress")) -> (error out=w400:errorcluster)  [unwired: 1 in, 1 out]
        n182 = Build Path(base path=w391, name or relative path=path "_Measurement Plugin Converter/Utilities/Sequence Creation/CreateSequence_Main.vi") -> (appended path=w389:path)
        n183 = case shown="True" w398 {
          tunnel: w389 -> [_ w421]
          tunnel: w402 -> [_ w417]
          tunnel: w401 -> [_ w416]
          tunnel: [w408 w411] -> w394
          tunnel: w400 -> [w408 w413]
          tunnel: ["" T7 "Create template measurement sequence" ("EventData.EventValues")] -> w393
          frame False {
          }
          frame True {
            n184 = Open VI Reference(type specifier VI Refnum (for type only)=refnum<vi> refnum, vi path=w421, options=256, error in (no error)=w413) -> (vi reference=w418:refnum<vi>, error out=w422:errorcluster)  [unwired: 2 in]
            n185 = call-by-ref "?"(reference=w418, error in=w422, "Project Path"=w417, "Measurement Name"=w416) -> (reference out=w414:refnum<vi>, error out=w420:errorcluster)  [unwired: 13 in, 1 out]
            n186 = Close Reference(reference=w414, error in (no error)=w420) -> (error out=w412:errorcluster)
            n187 = call "Set SubroutineInfo.vi"("Subroutine In"="Creating template teststand measurement sequence", "error in (no error)"=w412) -> ("error out"=w411:errorcluster)  [unwired: 13 in]
          }
        }
        n188 = Bundle By Name(cluster=w403, "EventData.EventValues"=w393) -> (w395:T3)
      }
      frame "Show Next Steps" {
        # "Open the LabVIEW project once conversion is complete"
        n189 = property on="Status" class="Str"(error in=w426, "Value"="Saving the Project and Libraries..." ("Status")) -> (error out=w424:errorcluster)  [unwired: 1 in, 1 out]
        n190 = property on="Progress" class="Slide (strict)"(error in=w424, "Value"=i8 96 ("Progress")) -> (error out=w423:errorcluster)  [unwired: 1 in, 1 out]
        n191 = call "Save Libraries and Projects.vi"("error in (no error)"=w423) -> ("error out"=w429:errorcluster)  [unwired: 10 in]
        n192 = property on="Tab Control" class="TabCtl (strict)"(error in=w429, "Value"=enum32{"User Inputs", "Progress", "Next Steps"}."Next Steps" ("Tab Control")) -> (error out=w428:errorcluster)  [unwired: 1 in, 1 out]
      }
      frame "Convert Next Module" {
        w432 = ""
        w433 = FALSE ("Module Data.Valid Code Path?")
        # "Reinitialize for the next conversion"
        n193 = property on="Tab Control" class="TabCtl (strict)"(error in=w437, "Value"=enum32{"User Inputs", "Progress", "Next Steps"}."User Inputs" ("Tab Control")) -> (error out=w434:errorcluster)  [unwired: 1 in, 1 out]
        n194 = property on="Create Measurement Service" class="Bool"(error in=w434, "DisabledEnum"=T2."Disabled and Grayed Out" ("Disabled")) -> (error out=w435:errorcluster)  [unwired: 1 in, 1 out]
        n195 = Bundle By Name(cluster=w441, "Input Data.Code Module"=path "", "Input Data.Measurement Name"=w432, "Module Data.Valid Code Path?"=w433, "Module Data.Valid Meas Name?"=w433, "Input Data.Description"=w432) -> (w440:T3)
      }
      frame "*******************************LOGGER**********************************" {
      }
      frame "Event Logger" {
        # "Logs the events of code conversion utility"
        n196 = Unbundle By Name(w447) -> ("EventData"=w446:T6)
        n197 = call "LogToFile.vi"("EventData in"=w446, "Error In"=w449) -> ("EventData out"=w444:T6, "Error Out"=w448:errorcluster)  [unwired: 12 in]
        n198 = Bundle By Name(cluster=w447, "EventData"=w444) -> (w445:T3)
      }
      frame "*******************************EXIT**********************************" {
      }
      frame "Exit" {
        # "Delete all the dictionaries"
        n199 = call "Queue Driver.vi"("error in (no error)"=w459, "Q Operations"=Queue_Operations."Flush") -> ("error out"=w457:errorcluster)  [unwired: 12 in, 1 out]
        n200 = call "Queue Driver.vi"("error in (no error)"=w457, "Q Operations"=Queue_Operations."Release") -> ("error out"=w454:errorcluster)  [unwired: 12 in, 1 out]
        n201 = call "Dictionary.vi"("error in (no error)"=w454, "Dict States"=Dictionary_States."Delete All") -> ("error out"=w453:errorcluster)  [unwired: 12 in, 1 out]
      }
      frame "***********************************ERROR**********************************" {
      }
      frame "Error" {
        # "Handle error"
        n202 = call <vilib>:"Clear Errors.vi"("error in (no error)"=w464) -> ("error out"=w466:errorcluster)  [unwired: 5 in, 1 out]
        n203 = call "Queue Driver.vi"("error in (no error)"=w466, "Q Operations"=Queue_Operations."Flush") -> ("error out"=w465:errorcluster)  [unwired: 12 in, 1 out]
        n204 = case shown="False" FALSE {
          tunnel: w465 -> [w471 w477]
          tunnel: [w470 w475] -> w469
          frame False {
            n205 = call "Queue Driver.vi"("States[]"=string[] ["Event Logger", "Convert Next Module", "Update FP Elements"], "error in (no error)"=w471, "Q Operations"=Queue_Operations."Enqueue N") -> ("error out"=w470:errorcluster)  [unwired: 11 in, 1 out]
          }
          frame True {
            n206 = call "Queue Driver.vi"("States[]"=string[] ["Cleanup", "Exit"], "error in (no error)"=w477, "Q Operations"=Queue_Operations."Enqueue N") -> ("error out"=w475:errorcluster)  [unwired: 11 in, 1 out]
          }
        }
      }
    }
  }
  n207 = invoke class="VI" method="FP.Close"(error in=w3) -> ()  [unwired: 2 in, 3 out]
  "Warning" <- TRUE ("Warning")
